vi "Build Assert VI Path.vi"(6 "Assert VI path":path, 7 "Type":T1, 8 "error in (no error)":errorcluster, 10 "Template Path":path) -> (0 "error out":errorcluster)   [LabVIEW 2018]
doc: "Creates a new vi based on the specified template and saves it to the new path"
uses:
  <vilib>/Utility/Data Type/Type Definitions/Data Type.ctl
  <vilib>/Utility/Data Type/NI_Data Type.lvlib
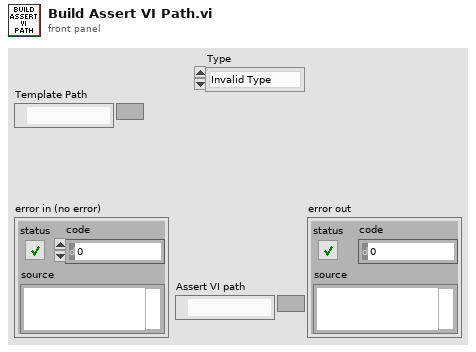
[diagram p1: front panel]
types:
  T1 = typedef "NI_Data Type.lvlib/Data Type.ctl" = enum8{"Invalid Type", "Void", "I8", "I16", "I32", "I64", "U8", "U16", "U32", "U64", "Single Float", "Double Float", "Extended Float", "Single Complex", "Double Complex", "Extended Complex", "Enum U8", "Enum U16", "Enum U32", "Enum U64", "Single Float With Unit", "Double Float With Unit", "Extended Float With Unit", "Single Complex with Unit", "Double Complex with Unit", "Extended Complex with Unit", "Boolean", "String", "Path", "Picture", "Tag", "Array", "Cluster", "Variant", "LV Variant", "Waveform", "Timestamp", "Digital Waveform", "Digital Data", "ExpressData", "Refnum", "External Data", "VI", "Poly VI", "LabVIEW Class Instance", "Fixed Point"}
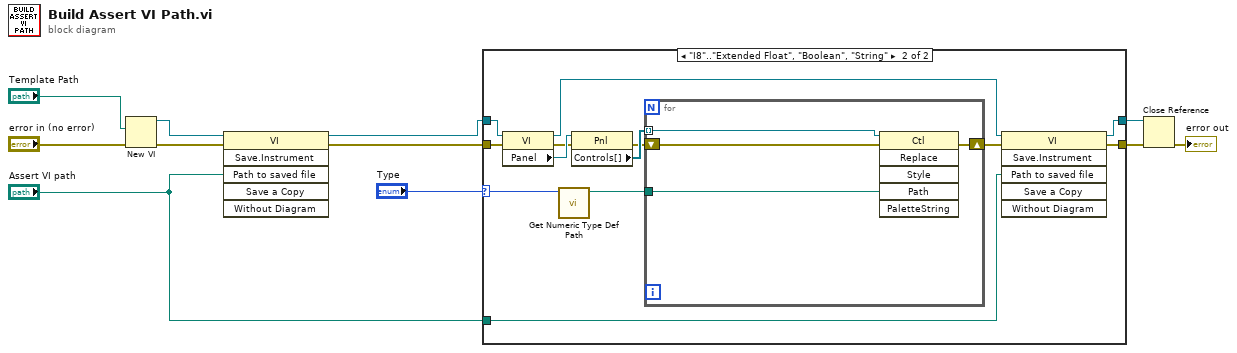
[diagram p0: block diagram]
diagram:
  n1 = New VI(8:"error in (no error)", 10:"Template Path") -> (0:w8:errorcluster, 3:w7:refnum<vi>)  [unwired: 5 in]
  n2 = invoke class="VI" method="Save.Instrument"(reference=w7, error in=w8, "Path to saved file"="Assert VI path") -> (reference out=w5:refnum<vi>, error out=w3:errorcluster)  [unwired: 3 in, 4 out]
  n3 = case shown="\"I8\"..\"Extended Float\", \"Boolean\", \"String\"" "Type" {
    selector: "Type" -> [_ w15]
    tunnel: [w13 w17] -> w6
    tunnel: w5 -> [w13 w26]
    tunnel: [w12 w19] -> w4
    tunnel: w3 -> [w12 w20]
    tunnel: "Assert VI path" -> [_ w16]
    frame Default {
    }
    frame "I8".."Extended Float", "Boolean", "String" {
      n4 = property class="VI"(reference=w26, error in=w20) -> (reference out=w18:refnum<vi>, error out=w21:errorcluster, "Panel"=w25:refnum<vi>)
      n5 = call "Get Numeric Type Def Path.vi"("Type"=w15) -> ("Numeric Type Def Path"=w14:path)  [unwired: 9 in, 1 out]
      n6 = property class="Pnl"(reference=w25, error in=w21) -> (error out=w22:errorcluster, "Controls[]"=w24:refnum<vi>[])  [unwired: 1 out]
      n7 = for {
        tunnel: w24 -> [w30] mode=indexing
        shift-right: [w29] -> w23
        shift-left: w22 -> [w28]
        tunnel: w14 -> [w27]
        n8 = invoke class="Ctl" method="Replace"(reference=w30, error in=w28, "Path"=w27) -> (error out=w29:errorcluster)  [unwired: 3 in, 5 out]
      }
      n9 = invoke class="VI" method="Save.Instrument"(reference=w18, error in=w23, "Path to saved file"=w16) -> (reference out=w17:refnum<vi>, error out=w19:errorcluster)  [unwired: 3 in, 4 out]
    }
  }
  n10 = Close Reference(reference=w6, error in (no error)=w4) -> (error out=→"error out":errorcluster)
